vi "Configure Event Input.vi"(7 "Detected Edge (0: Falling)":i32(ring) items=["Falling", "Rising", "Either"], 8 "error in (no error)":errorcluster, 10 "Input Source (0: Digital 1)":i32(ring) items=["Digital 1"=0, "Digital 2"=1, "Digital 3"=2, "Digital 4"=3, "Digital 5"=4, "Digital 6"=5, "Lan 1"=10, "Lan 2"=11, "Lan 3"=12, "Lan 4"=13, "Lan 5"=14, "Lan 6"=15, "Lan 7"=16, "Lan 8"=17, "External In"=18], 11 "VISA resource name":refnum<visa-resource-name>) -> (0 "error out":errorcluster, 3 "VISA resource name out":refnum<visa-resource-name>)   [LabVIEW 2015, in "Keithley DMM6500 DAQ6500 Series.lvlib"]
doc: "Sets the trigger operation and detection mode of the specified event."
uses:
  <instrlib>/Keithley DMM6500 DAQ6500 Series/Keithley DMM6500 DAQ6500 Series.lvlib
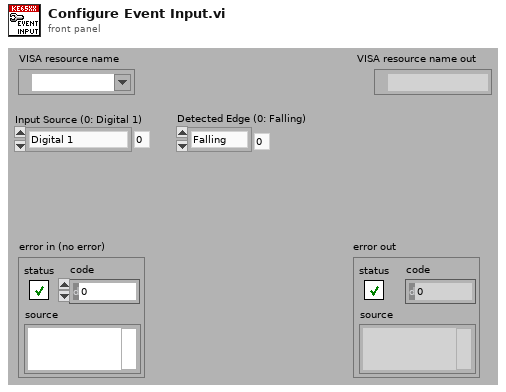
[diagram p1: front panel]
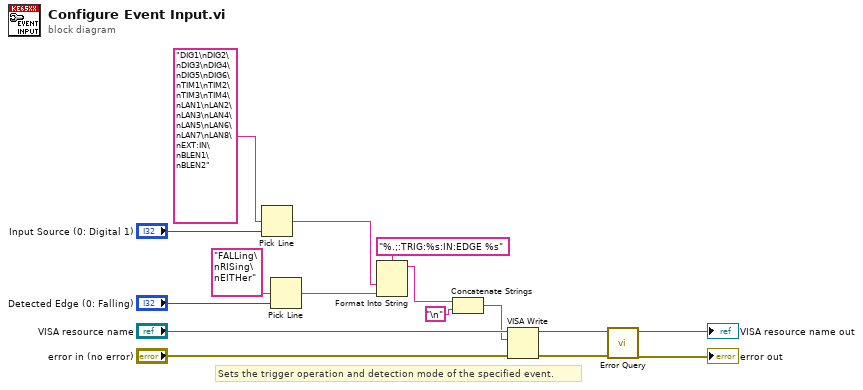
[diagram p0: block diagram]
diagram:
  # "Sets the trigger operation and detection mode of the specified event."
  n1 = Pick Line(multi-line string="DIG1\nDIG2\nDIG3\nDIG4\nDIG5\nDIG6\nTIM1\nTIM2\nTIM3\nTIM4\nLAN1\nLAN2\nLAN3\nLAN4\nLAN5\nLAN6\nLAN7\nLAN8\nEXT:IN\nBLEN1\nBLEN2", line index="Input Source (0: Digital 1)") -> (output string=w13:string)  [unwired: 1 in]
  n2 = Pick Line(multi-line string="FALLing\nRISing\nEITHer", line index="Detected Edge (0: Falling)") -> (output string=w4:string)  [unwired: 1 in]
  n3 = Format Into String(format string="%.;:TRIG:%s:IN:EDGE %s", w13, w4) -> (resulting string=w2:string)  [unwired: 2 in, 1 out]
  n4 = Concatenate Strings(w2, "\n") -> (w3:string)
  n5 = VISA Write(VISA resource name="VISA resource name", write buffer=w3, error in (no error)="error in (no error)") -> (VISA resource name out=w10:refnum<visa-resource-name>, error out=w9:errorcluster)  [unwired: 1 out]
  n6 = call <instrlib>:"Error Query.vi"("error in (no error)"=w9, "VISA resource name"=w10) -> ("error out"=→"error out":errorcluster, "VISA resource name out"=→"VISA resource name out":refnum<visa-resource-name>)  [unwired: 6 in, 2 out]
